vi "Teleop.vi"(10 "Match Info":T1={"Autonomous Elapsed Seconds"=0.0, "TeleOp Elapsed Seconds"=0.0, "Disabled Elapsed Seconds"=0.0, "Visited Autonomous"=FALSE, "Visited TeleOp"=FALSE, "Visited Disabled"=FALSE, "Autonomous Settings"={"Autonomous Style"=enum."Independent", "VI Refnum"=refnum}}, 11 "Call Context":T2) -> ()   [LabVIEW 2018]
doc: "This VI is called for each TeleOp packet received from the DS where the robot is not disabled. It is often used to read from the joysticks and update I/O or to update setpoints for timed control loops. It should complete and return within 20 milliseconds or it may miss DS packets."
uses:
  <vilib>/Rock Robotics/WPI/DriverStation/WPI_DriverStationDerivedRobotMode.ctl
  <vilib>/Rock Robotics/WPI/DriverStation/WPI_DriverStationMatch Info.ctl
  RobotGlobal.vi
  Classes/Drive/Drive.lvclass
  Classes/Pnematics control/Pneumatics.lvclass
  Classes/Joysticks/Joysticks.lvclass
  Classes/Elevator/Elevator.lvclass
  Classes/Hatch/Hatch.lvclass
  Classes/Cargo/Cargo.lvclass
  Classes/Pnematics control/Solenoids/Solenoids.lvclass
  Classes/Vision/Vision.lvclass
panel:
  out "error out":errorcluster
  in  "error in (no error)":errorcluster
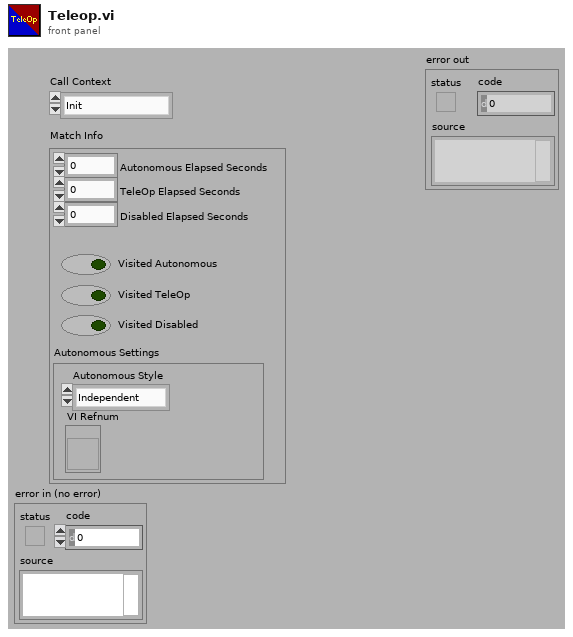
[diagram p1: front panel]
types:
  T1 = typedef "WPI_DriverStationMatch Info.ctl" = cluster{"Autonomous Elapsed Seconds":dbl, "TeleOp Elapsed Seconds":dbl, "Disabled Elapsed Seconds":dbl, "Visited Autonomous":bool, "Visited TeleOp":bool, "Visited Disabled":bool, "Autonomous Settings":cluster{"Autonomous Style":enum16{"Iterative", "Independent"}, "VI Refnum":refnum<vi>}}
  T2 = typedef "WPI_DriverStationDerivedRobotMode.ctl" = enum16{"Init", "Execute", "Stop"}
  T3 = typedef "RobotObjects.ctl" = cluster{"Drive.lvclass":refnum<class "Drive.lvclass">, "Pneumatics.lvclass":refnum<class "Pneumatics.lvclass">, "Vision.lvclass":refnum<class "Vision.lvclass">, "Joysticks.lvclass":refnum<class "Joysticks.lvclass">, "Elevator.lvclass":refnum<class "Elevator.lvclass">, "Hatch.lvclass":refnum<class "Hatch.lvclass">, "Cargo.lvclass":refnum<class "Cargo.lvclass">}
  T4 = typedef "Joysticks.lvlib/Joysticks.lvclass/JoystickData.ctl" = cluster{"X Axis":dbl, "Y Axis":dbl, "Drivetrain Shifter (Hold)":bool, "Beak (Toggle)":bool, "Cargo In (Hold)":bool, "Cargo Out (Hold)":bool, "Switch to hatch(toggle)":bool, "Switch to cargo(toggle)":bool, "Elevator Up (Toggle)":bool, "Elevator Down (Toggle)":bool, "AutoForward (Hold)":bool, "Climb(toggle)":bool, "Disengage Climb(toggle)":bool, "AutoTurn(hold)":bool, "CamMode(Two Driver only)":bool, "AltPipeline":bool}
  T5 = typedef "Pneumatics control.lvlib/Pneumatics.lvclass/Solenoids.ctl" = cluster{"DriveShift":refnum<class "Solenoids.lvclass">, "ArmLock":refnum<class "Solenoids.lvclass">, "HatchArm":refnum<class "Solenoids.lvclass">, "HatchGrabber":refnum<class "Solenoids.lvclass">}
  T6 = typedef "Elevator.lvlib/Elevator.lvclass/Elevator Position.ctl" = enum16{"C0, Cargo Ground", "C1, LV1 Cargo", "C2, Cargo Ship Cargo", "H0, LV1 Hatch", "H1, LV2 Hatch"}
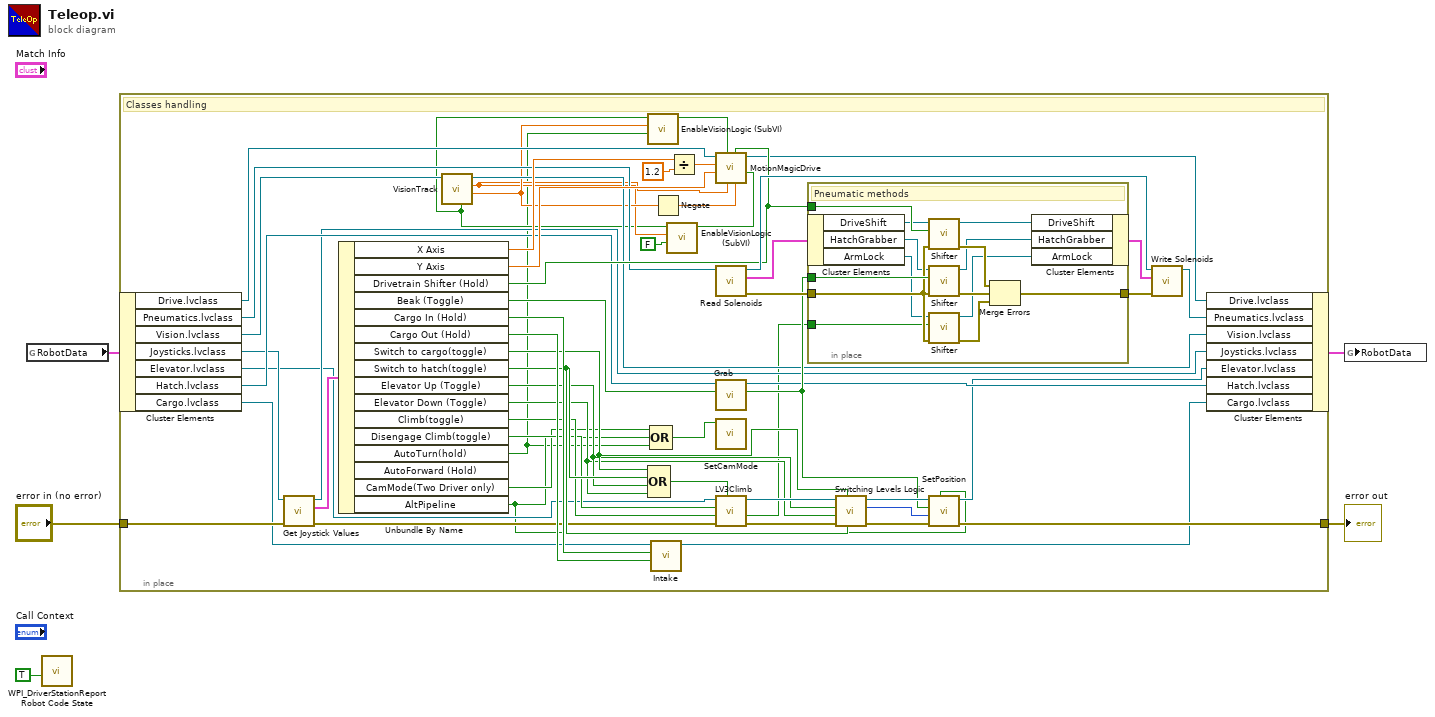
[diagram p0: block diagram]
diagram:
  n1 = global read "RobotGlobal.vi" "RobotData"() -> (w3:T3)
  n2 = call <vilib>:"WPI_DriverStationReport Robot Code State.vi"("TeleOp"=TRUE ("Autonomous")) -> ()  [unwired: 10 in, 1 out]
  n3 = in-place {
    in-place-border: "error in (no error)" -> [w38]
    in-place-border: [w34] -> w1
    # "Classes handling"
    n4 = in-place-cluster #1(w3) -> ("Drive.lvclass"=w56:refnum<class "Drive.lvclass">, "Pneumatics.lvclass"=w27:refnum<class "Pneumatics.lvclass">, "Vision.lvclass"=w25:refnum<class "Vision.lvclass">, "Joysticks.lvclass"=w23:refnum<class "Joysticks.lvclass">, "Elevator.lvclass"=w21:refnum<class "Elevator.lvclass">, "Hatch.lvclass"=w29:refnum<class "Hatch.lvclass">, "Cargo.lvclass"=w31:refnum<class "Cargo.lvclass">)
    n5 = call-dynamic "Get Joystick Values.vi"("error in (no error)"=w38, "Joysticks in"=w23) -> ("error out"=w40:errorcluster, "Joystick Data"=w39:T4, "Joysticks out"=w22:refnum<class "Joysticks.lvclass">)  [unwired: 7 in]
    n6 = Unbundle By Name(w39) -> ("X Axis"=w52:dbl, "Y Axis"=w51:dbl, "Drivetrain Shifter (Hold)"=w50:bool, "Beak (Toggle)"=w49:bool, "Cargo In (Hold)"=w48:bool, "Cargo Out (Hold)"=w47:bool, "Switch to cargo(toggle)"=w46:bool, "Switch to hatch(toggle)"=w45:bool, "Elevator Up (Toggle)"=w44:bool, "Elevator Down (Toggle)"=w43:bool, "Climb(toggle)"=w42:bool, "Disengage Climb(toggle)"=w41:bool, "AutoTurn(hold)"=w6:bool, "CamMode(Two Driver only)"=w9:bool, "AltPipeline"=w7:bool)  [unwired: 1 out]
    n7 = call "VisionTrack.vi"("Vision in"=w25) -> ("VerticalOffset(degrees)"=w16:dbl, "HorizontalOffset(degrees)"=w14:dbl, "Vision out"=w24:refnum<class "Vision.lvclass">, "Target?"=w12:bool)  [unwired: 5 in, 2 out]
    n8 = call "EnableVisionLogic (SubVI).vi"("Activate?(hold)"=w6, "Offset(degrees)"=w16, "Target?"=w12) -> ("Enable?"=w15:bool)  [unwired: 8 in]
    n9 = Compound Arithmetic op=OR(w46, w45, w44, w43) -> (w53:bool)
    n10 = Compound Arithmetic op=OR(w9, w7, w6) -> (w8:bool)
    n11 = call-dynamic "Intake.vi"("Out"=w47, "In"=w48, "Cargo in"=w31) -> ("Cargo out"=w30:refnum<class "Cargo.lvclass">)  [unwired: 7 in, 1 out]
    n12 = Negate(x=w16) -> (-x=w11:dbl)
    n13 = call "EnableVisionLogic (SubVI).vi"("Activate?(hold)"=FALSE, "Offset(degrees)"=w14, "Target?"=w12) -> ("Enable?"=w13:bool)  [unwired: 8 in]
    n14 = Divide(x=w52, y=1.2) -> (x/y=w18:dbl)
    n15 = call-dynamic "MotionMagicDrive.vi"("Enable Vision Y"=w13, "X offset"=w11, "High gear?"=w50, "Y offset"=w14, "Enable Vision X"=w15, "Y Axis"=w51, "X Axis"=w18, "Drive in"=w56) -> ("Drive out"=w32:refnum<class "Drive.lvclass">)  [unwired: 2 in, 1 out]
    n16 = call-dynamic "Read Solenoids.vi"("Pneumatics in"=w27) -> ("error out"=w59:errorcluster, "Solenoids"=w58:T5, "Pneumatics out"=w57:refnum<class "Pneumatics.lvclass">)  [unwired: 8 in]
    n17 = call-dynamic "Grab.vi"("Grab Toggle?"=w49, "Hatch in"=w29) -> ("Solenoid On?"=w33:bool, "Hatch out"=w28:refnum<class "Hatch.lvclass">)  [unwired: 7 in, 1 out]
    n18 = call "SetCamMode.vi"("Normal camera?"=w8) -> ()  [unwired: 11 in]
    n19 = call-dynamic "LV3Climb.vi"("Deactivate?"=w53, "error in (no error)"=w40, "Activate?"=w42, "Redeploy?"=w41, "Elevator in"=w21) -> ("error out"=w55:errorcluster, "activate wrist lock"=w19:bool, "Elevator out"=w54:refnum<class "Elevator.lvclass">)  [unwired: 4 in]
    n20 = in-place {
      in-place-border: w50 -> [w74]
      in-place-border: w59 -> [w68]
      in-place-border: [w72] -> w61
      in-place-border: w33 -> [w70]
      in-place-border: w19 -> [w67]
      # "Pneumatic methods"
      n21 = in-place-cluster #2(w58) -> ("DriveShift"=w66:refnum<class "Solenoids.lvclass">, "HatchGrabber"=w65:refnum<class "Solenoids.lvclass">, "ArmLock"=w64:refnum<class "Solenoids.lvclass">)
      n22 = call-dynamic "Shifter.vi"("error in (no error)"=w68, "Solenoid On?"=w74, "Solenoids in"=w66) -> ("error out"=w73:errorcluster, "Solenoids out"=w75:refnum<class "Solenoids.lvclass">)  [unwired: 7 in]
      n23 = call-dynamic "Shifter.vi"("error in (no error)"=w68, "Solenoid On?"=w70, "Solenoids in"=w65) -> ("error out"=w71:errorcluster, "Solenoids out"=w63:refnum<class "Solenoids.lvclass">)  [unwired: 7 in]
      n24 = call-dynamic "Shifter.vi"("error in (no error)"=w68, "Solenoid On?"=w67, "Solenoids in"=w64) -> ("error out"=w69:errorcluster, "Solenoids out"=w62:refnum<class "Solenoids.lvclass">)  [unwired: 7 in]
      n25 = Merge Errors(w73, w71, w69) -> (w72:errorcluster)
      n26 = in-place-cluster #2("DriveShift"=w75, "HatchGrabber"=w63, "ArmLock"=w62) -> (w60:T5)
    }
    n27 = call "Switching Levels Logic.vi"("Hatch"=w45, "Cargo"=w46, "error in (no error)"=w55, "Down"=w43, "Up"=w44, "Elevator in"=w54) -> ("error out"=w37:errorcluster, "Cargo/Hatch"=w36:T6, "Elevator out"=w35:refnum<class "Elevator.lvclass">)  [unwired: 3 in]
    n28 = call-dynamic "SetPosition.vi"("AltPipe?"=w7, "error in (no error)"=w37, "Position"=w36, "Hach Grabed?"=w33, "Elevator in"=w35) -> ("error out"=w34:errorcluster, "Elevator out"=w20:refnum<class "Elevator.lvclass">)  [unwired: 5 in]
    n29 = call-dynamic "Write Solenoids.vi"("error in (no error)"=w61, "Solenoids"=w60, "Pneumatics in"=w57) -> ("Pneumatics out"=w26:refnum<class "Pneumatics.lvclass">)  [unwired: 7 in, 1 out]
    n30 = in-place-cluster #1("Drive.lvclass"=w32, "Pneumatics.lvclass"=w26, "Vision.lvclass"=w24, "Joysticks.lvclass"=w22, "Elevator.lvclass"=w20, "Hatch.lvclass"=w28, "Cargo.lvclass"=w30) -> (w4:T3)
  }
  "error out" <- w1
  n31 = global write "RobotGlobal.vi" "RobotData"(w4) -> ()
